vi "6.4.vi"   [LabVIEW 2017]
uses:
  <vilib>/Utility/file.llb/Write Delimited Spreadsheet (string).vi
  <vilib>/measure/NI_MABase.lvlib
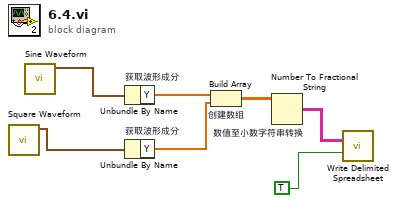
[diagram p0: block diagram]
diagram:
  n1 = call <vilib>:"Square Waveform.vi"() -> ("signal out"=w7:waveform(dbl))  [unwired: 10 in, 1 out]
  n2 = call <vilib>:"Sine Waveform.vi"() -> ("signal out"=w6:waveform(dbl))  [unwired: 10 in, 1 out]
  n3 = Unbundle By Name "获取波形成分"(w6) -> ("Y"=w5:dbl[])
  n4 = Unbundle By Name "获取波形成分"(w7) -> ("Y"=w4:dbl[])
  n5 = Build Array "创建数组"(w5, w4) -> (w3:dbl[][])
  n6 = Number To Fractional String "数值至小数字符串转换"(number=w3) -> (F-format string=w2:string[][])  [unwired: 3 in]
  n7 = call-poly <vilib>:"Write Delimited Spreadsheet.vi"("2D data"=w2, "append to file? (new file:F)"=TRUE) -> ()  [unwired: 12 in, 2 out]
